vi "Math-Uniform Random Number (I32, 2x1D).vi"(4 "N":i32, 5 "Ymax":i32, 6 "Xmax":i32) -> (1 "Yi":i32[](array[numeric]), 2 "Xi":i32[](array[numeric]))   [LabVIEW 2020]
uses:
  LinSpace (start-stop-step).vi
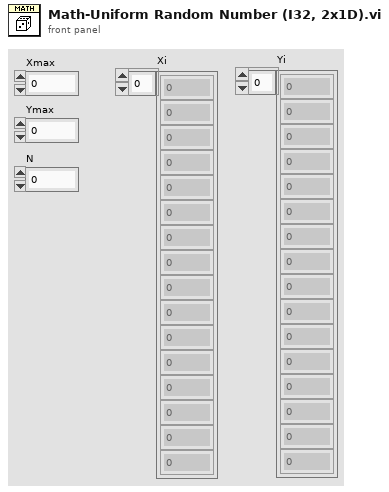
[diagram p1: front panel]
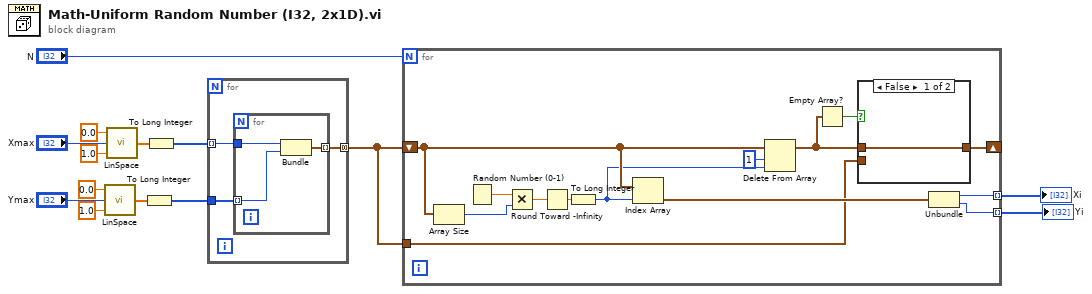
[diagram p0: block diagram]
diagram:
  n1 = call-poly "LinSpace.vi"("Step"=1.0, "Stop"="Ymax", "Start"=0.0) -> ("Array"=w12:dbl[])  [unwired: 1 in, 1 out]
  n2 = call-poly "LinSpace.vi"("Step"=1.0, "Stop"="Xmax", "Start"=0.0) -> ("Array"=w9:dbl[])  [unwired: 1 in, 1 out]
  n3 = To Long Integer(number=w12) -> (32bit integer=w5:i32[])
  n4 = To Long Integer(number=w9) -> (32bit integer=w4:i32[])
  n5 = for {
    tunnel: w5 -> [w16]
    tunnel: w4 -> [w17] mode=indexing
    tunnel: [w15] -> w1 mode=concatenating
    n6 = for {
      tunnel: w17 -> [w20]
      tunnel: w16 -> [w19] mode=indexing
      tunnel: [w18] -> w15 mode=indexing
      n7 = Bundle("Numeric"=w20, "Numeric"=w19) -> (w18:cluster{"Numeric":i32, "Numeric":i32})  [unwired: 1 in]
    }
  }
  n8 = for {
    N: "N" -> [_]
    shift-right: [w22] -> _
    shift-left: w1 -> [w30]
    tunnel: [w26] -> w3 mode=indexing
    tunnel: [w25] -> w2 mode=indexing
    tunnel: w1 -> [w21]
    n9 = Array Size(array=w30) -> (size(s)=w31:i32)
    n10 = Random Number (0-1)() -> (number: 0 to 1=w34:dbl)
    n11 = Multiply(x=w34, y=w31) -> (x*y=w33:dbl)
    n12 = Round Toward -Infinity(1:w33) -> (0:w32:dbl)
    n13 = To Long Integer(number=w32) -> (32bit integer=w28:i32)
    n14 = Index Array(array=w30, index=w28) -> (element=w29:cluster{"Numeric":i32, "Numeric":i32})
    n15 = Delete From Array(array=w30, length=1, index=w28) -> (array with subset deleted=w23:cluster{"Numeric":i32, "Numeric":i32}[])  [unwired: 1 out]
    n16 = Empty Array?(array=w23) -> (empty?=w24:bool)
    n17 = case shown="False" w24 {
      tunnel: w23 -> [w35 _]
      tunnel: [w35 w36] -> w22
      tunnel: w21 -> [_ w36]
      frame False {
      }
      frame True {
      }
    }
    n18 = Unbundle(w29) -> ("Numeric"=w26:i32, "Numeric"=w25:i32)
  }
  "Xi" <- w3
  "Yi" <- w2
